vi "一体站氨氮总磷流程质控自动启动.vi"(6 "CODMn量程切换":enum32{"H", "L", "AUTO"}(ring)=enum."AUTO", 8 "总磷量程切换":enum32{"H", "L", "AUTO"}(ring)=enum."AUTO", 9 "总氮量程切换":enum32{"H", "L", "AUTO"}(ring)=enum."AUTO", 10 "氨氮量程切换":enum32{"H", "L", "AUTO"}(ring)=enum."AUTO", 11 "参数":T1={"是否启用仪器"=FALSE, "CODMn"={"启动测量模式"={"测量模式"=enum."水样测量"}, "确定按钮"=TRUE}, "启动模块"={"氨氮"=FALSE, "总磷"=FALSE, "总氮"=FALSE, "CODMn"=FALSE, "CODCr"=FALSE}, "常规启动"=FALSE, "直接启动"=FALSE}) -> ()   [LabVIEW 2016, in "质控单元.lvlib"]
panel:
  out "枚举 2":enum16{"初始化", "采配水启动", "等待", "配水", "排水", "结束"}(ring)
  out "枚举":enum16{"初始化", "采配水启动", "等待", "配水", "排水", "结束"}(ring)
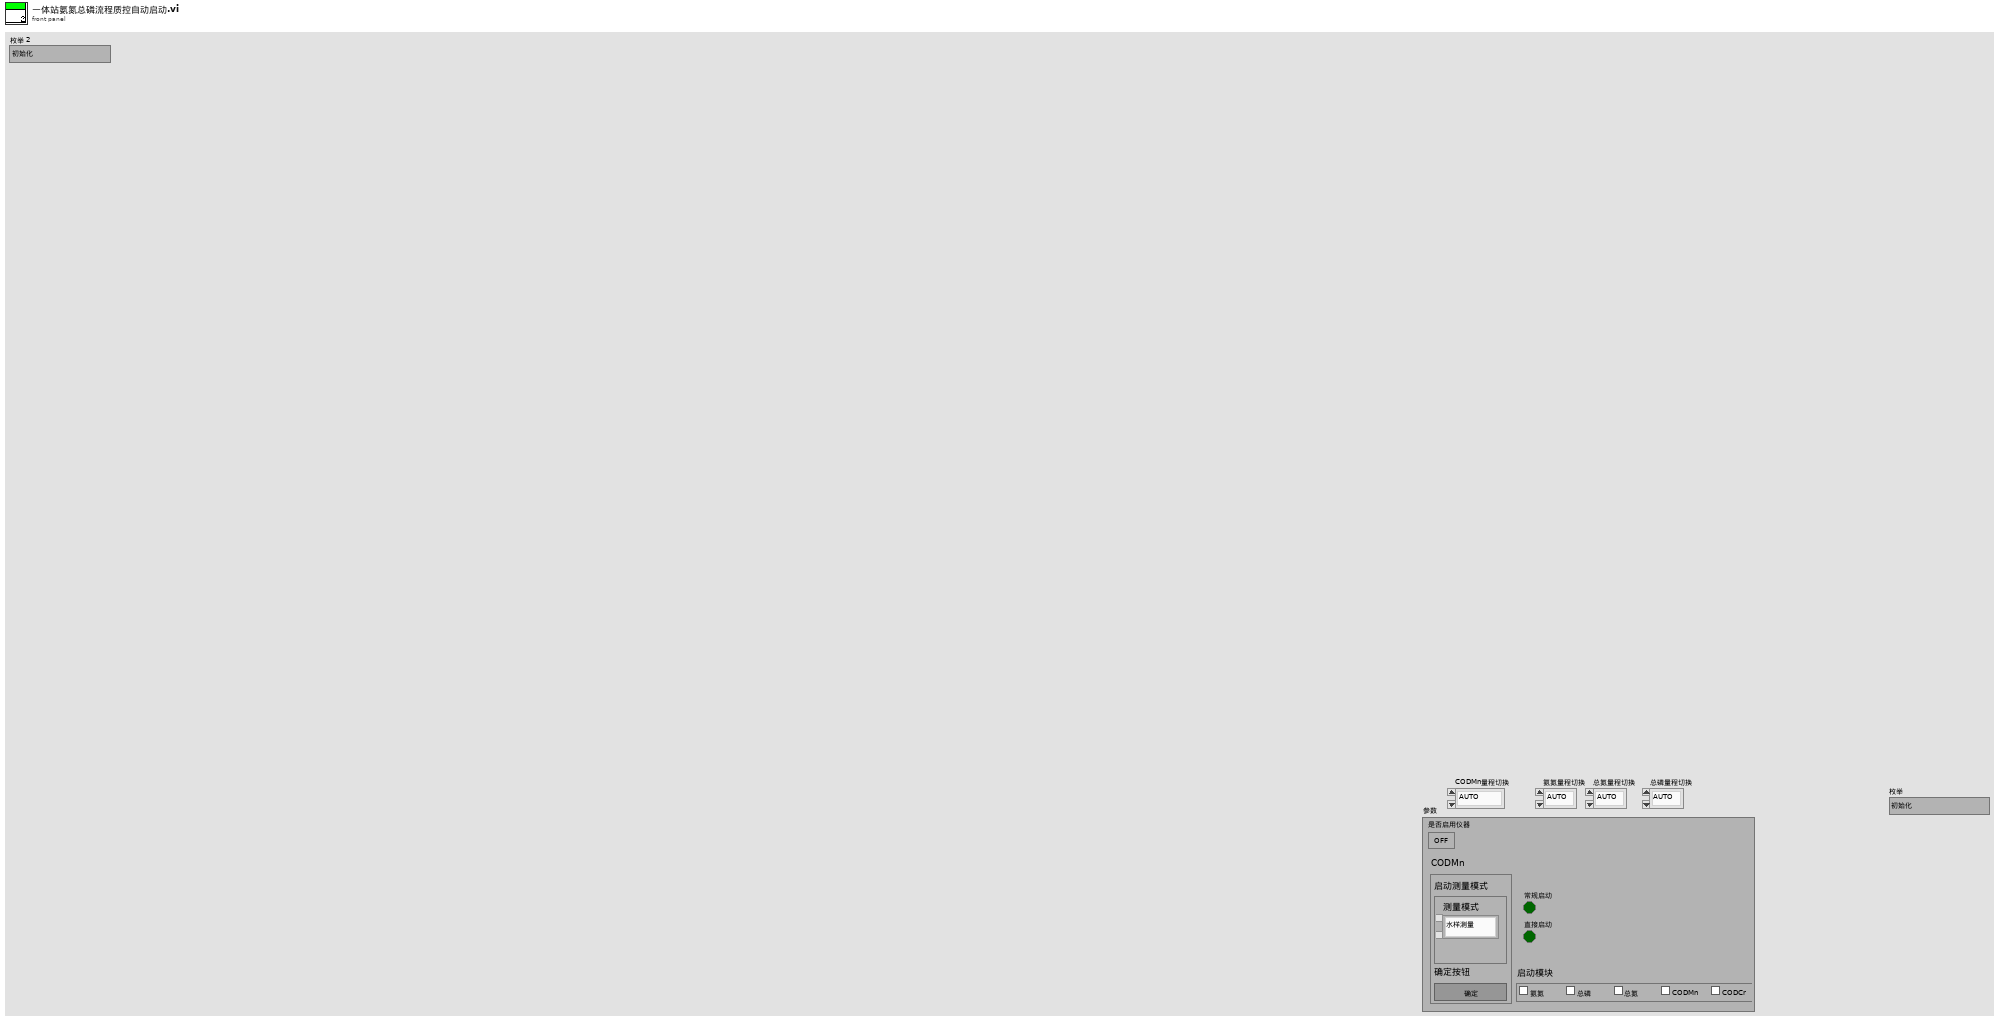
[diagram p1: front panel]
types:
  T1 = cluster{"是否启用仪器":bool, "CODMn":cluster{"启动测量模式":cluster{"测量模式":enum16{"水样测量", "标样核查", "加标回收", "平行样", "校零", "校标"}}, "确定按钮":bool}, "启动模块":cluster{"氨氮":bool, "总磷":bool, "总氮":bool, "CODMn":bool, "CODCr":bool}, "常规启动":bool, "直接启动":bool}
  T2 = cluster{"命令":string, cluster{"starting address":u16, "holding register value":u16}}
  T3 = cluster{"R0":i16, "R1":i16, "R2":i16, "R3":i16, "R4":i16, "R5":i16, "R6":i16, "R7":i16, "R8":i16, "R9":i16, "R10":i16, "R11":i16, "R12":i16, "R13":i16, "R14":i16, "R15":i16, "R16":i16, "R17":i16, "R18":i16, "R19":i16, "R20":i16, "R21":i16, "R22":i16, "R23":i16, "R24":i16, "R25":i16, "R26":i16, "R27":i16, "R28":i16, "R29":i16, "R30":i16, "R31":i16, "R32":i16, "R33":i16, "R34":i16, "R35":i16, "R36":i16, "R37":i16, "R38":i16, "R39":i16, "R40":i16, "R41":i16, "R42":i16, "R43":i16, "R44":i16, "R45":i16, "R46":i16, "R47":i16, "R48":i16, "R49":i16, "R50":i16, "R51":i16, "R52":i16, "R53":i16, "R54":i16, "R55":i16, "R56":i16}
  T4 = enum32{"Bad", "Idle", "Run top level", "Running"}
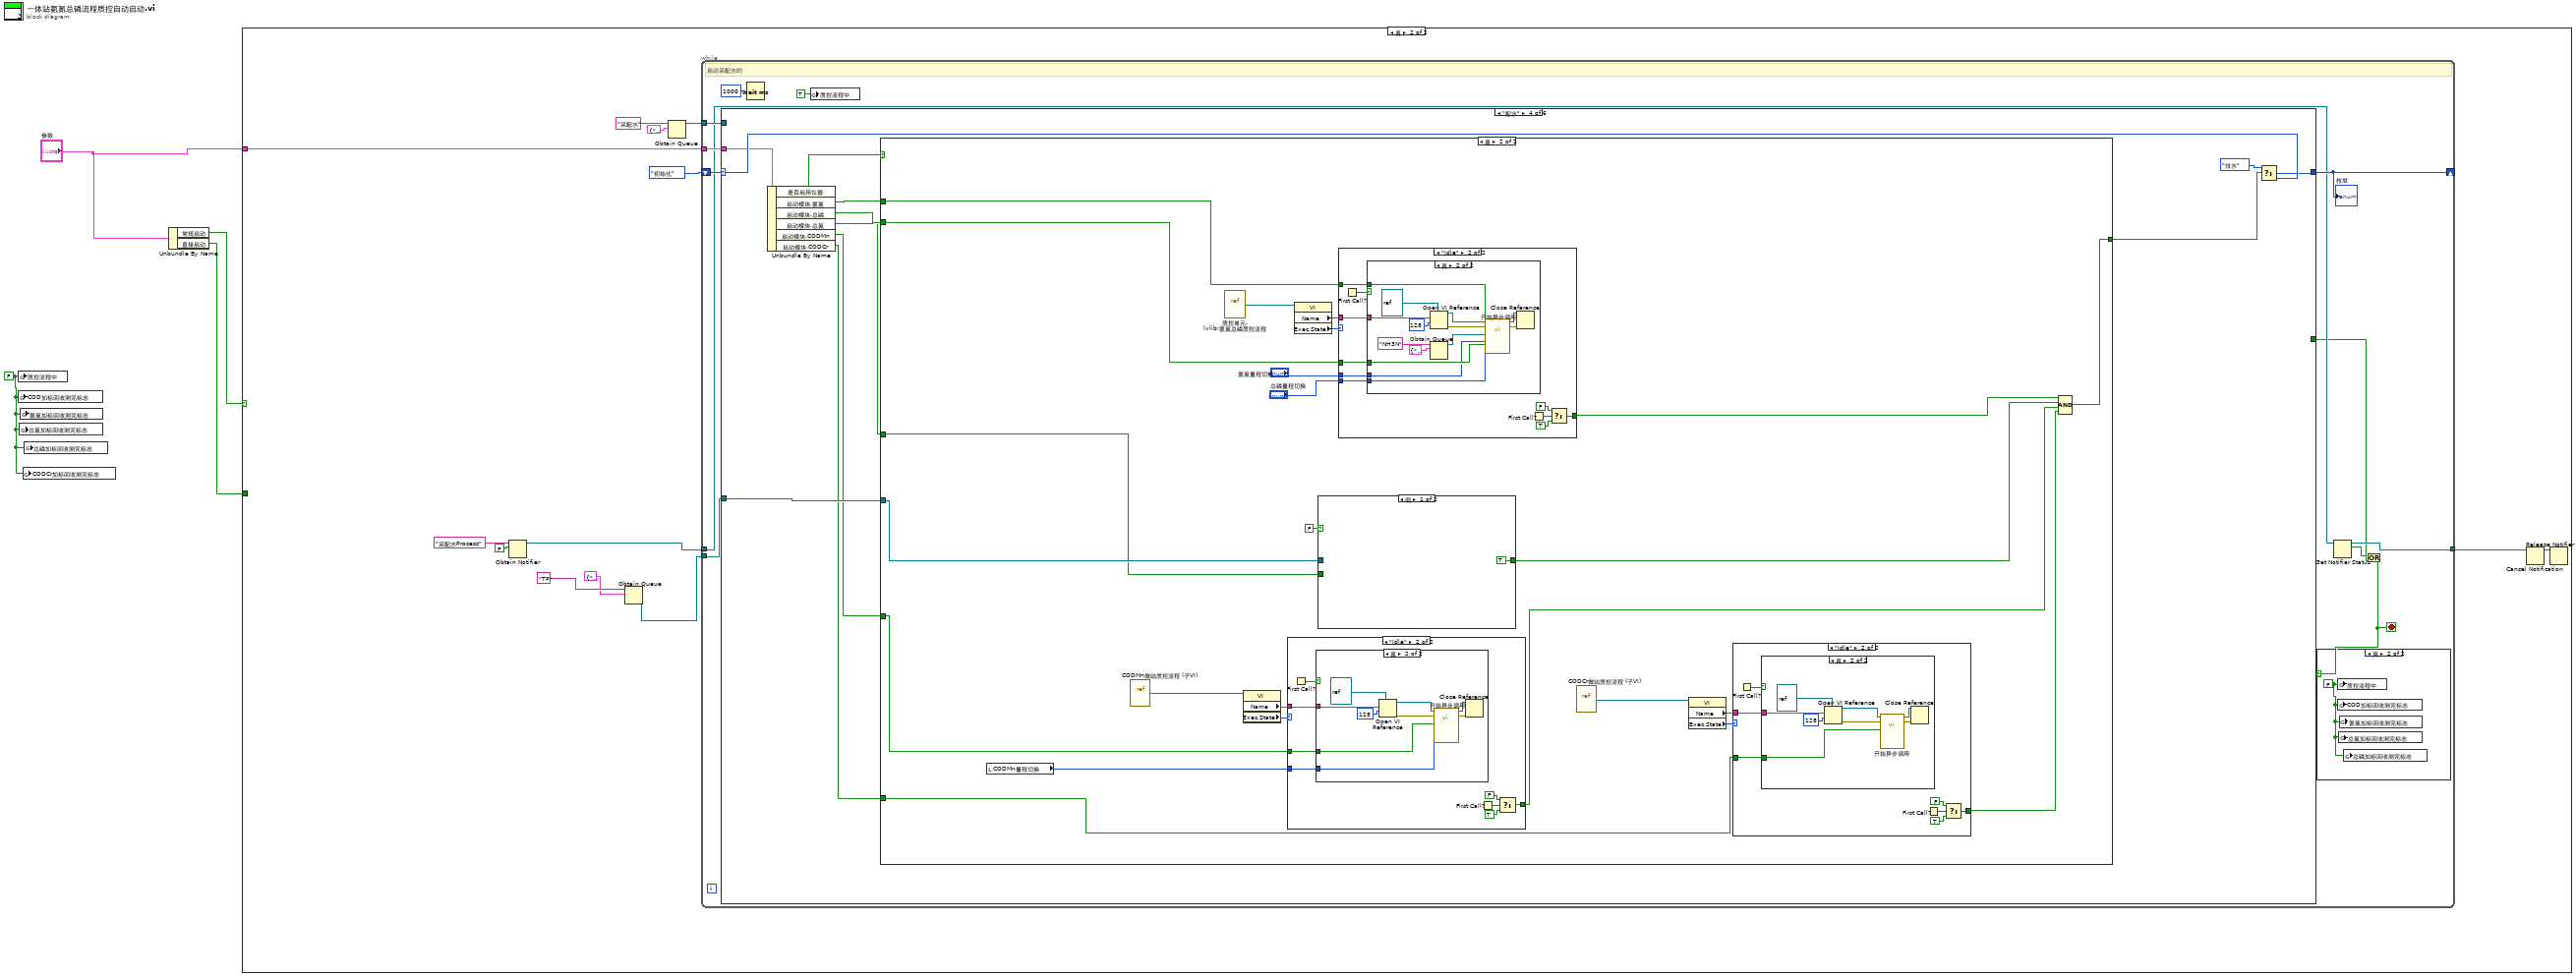
[diagram p0: block diagram]
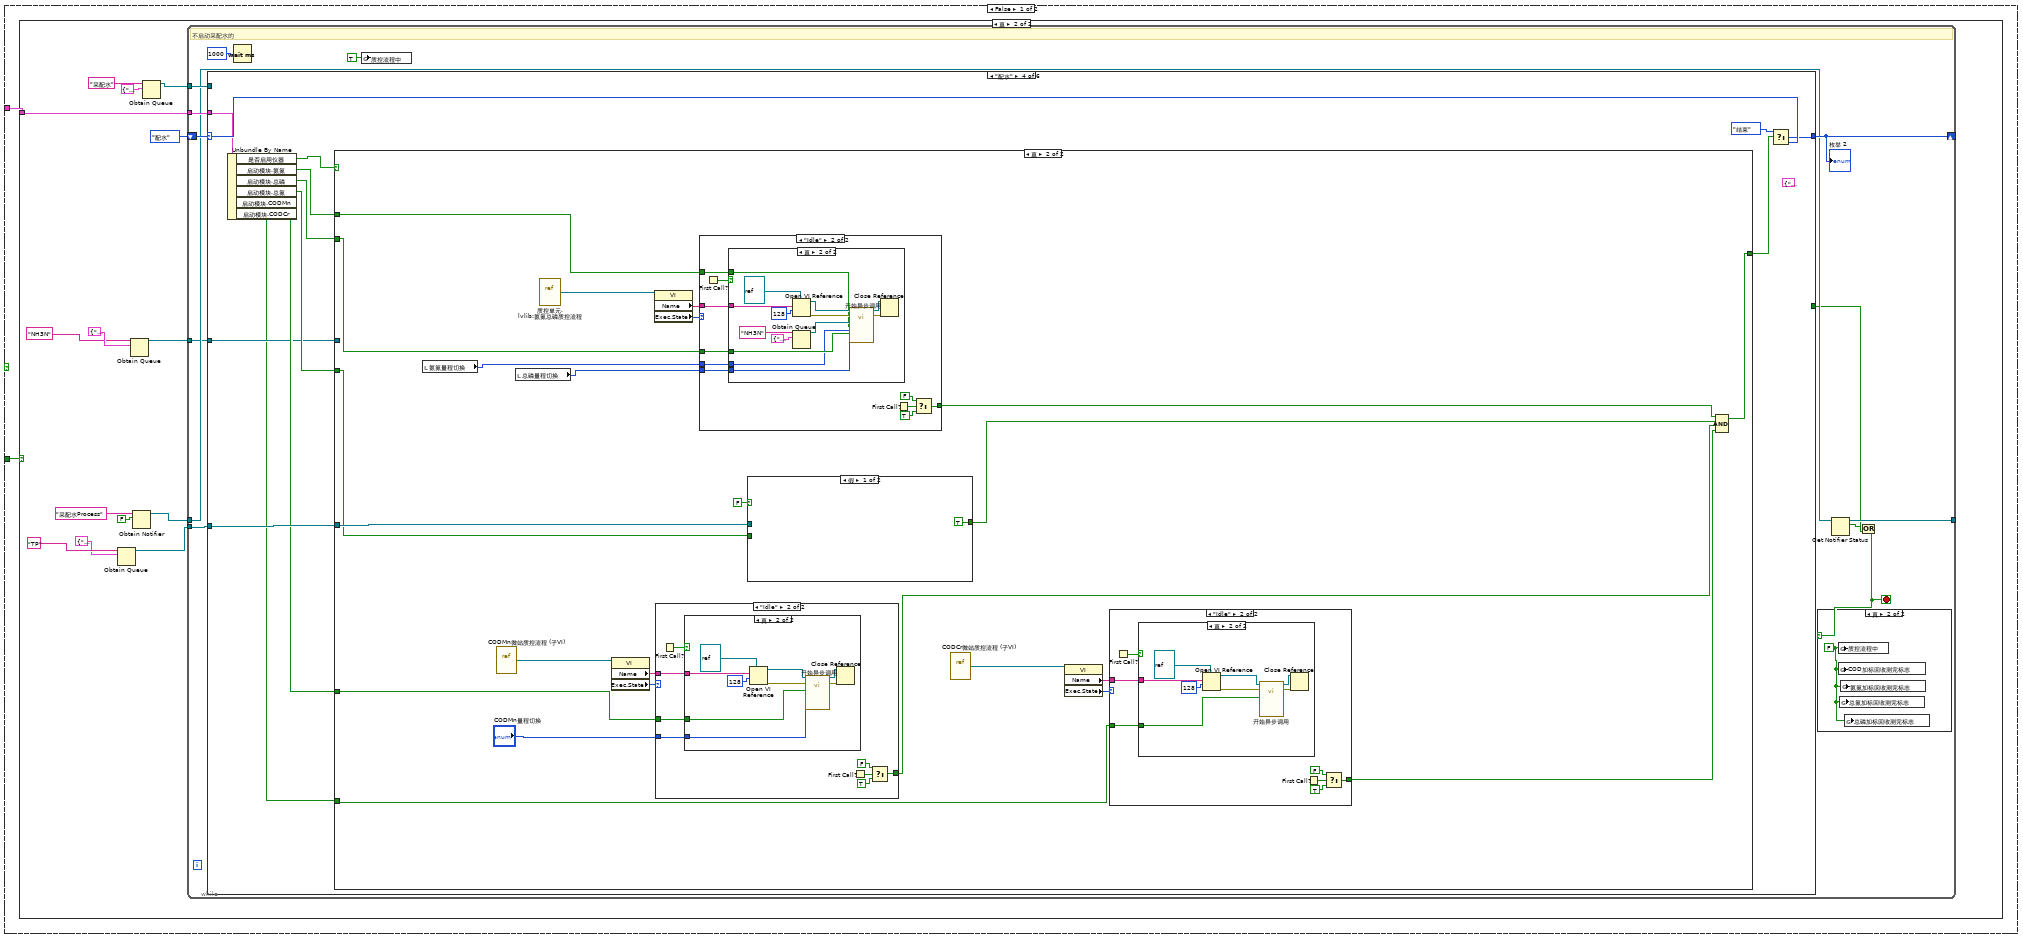
[diagram p2: hidden frame]
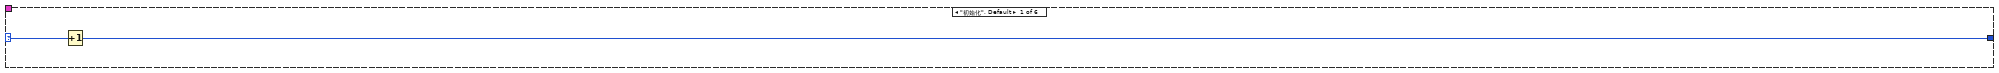
[diagram p5: hidden frame]
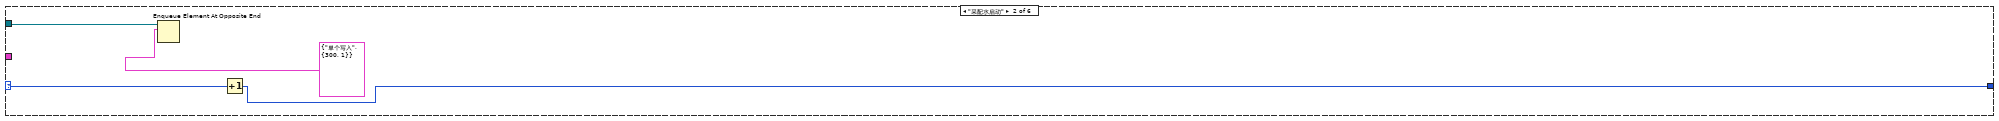
[diagram p6: hidden frame]
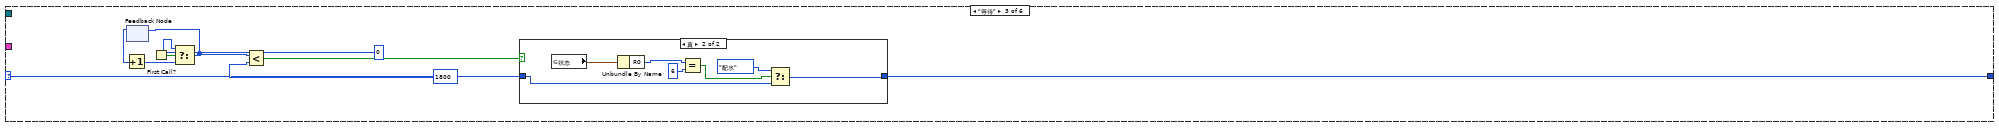
[diagram p7: hidden frame]
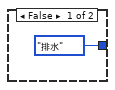
[diagram p8: hidden frame]
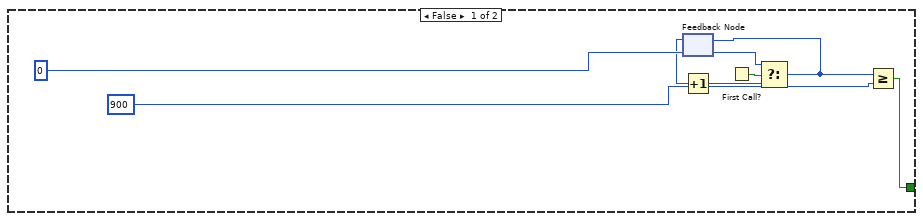
[diagram p9: hidden frame]
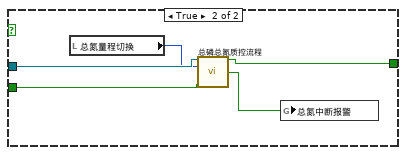
[diagram p16: hidden frame]
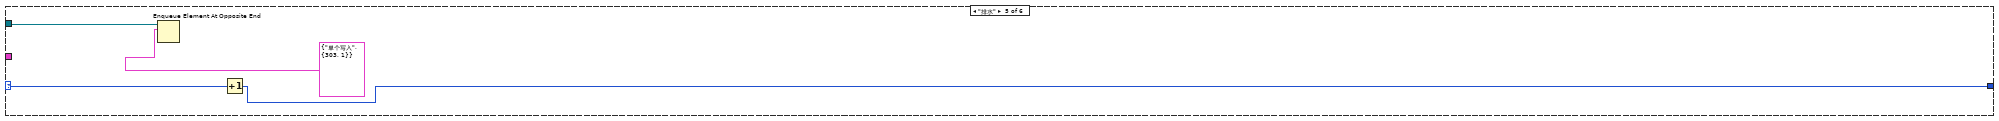
[diagram p17: hidden frame]
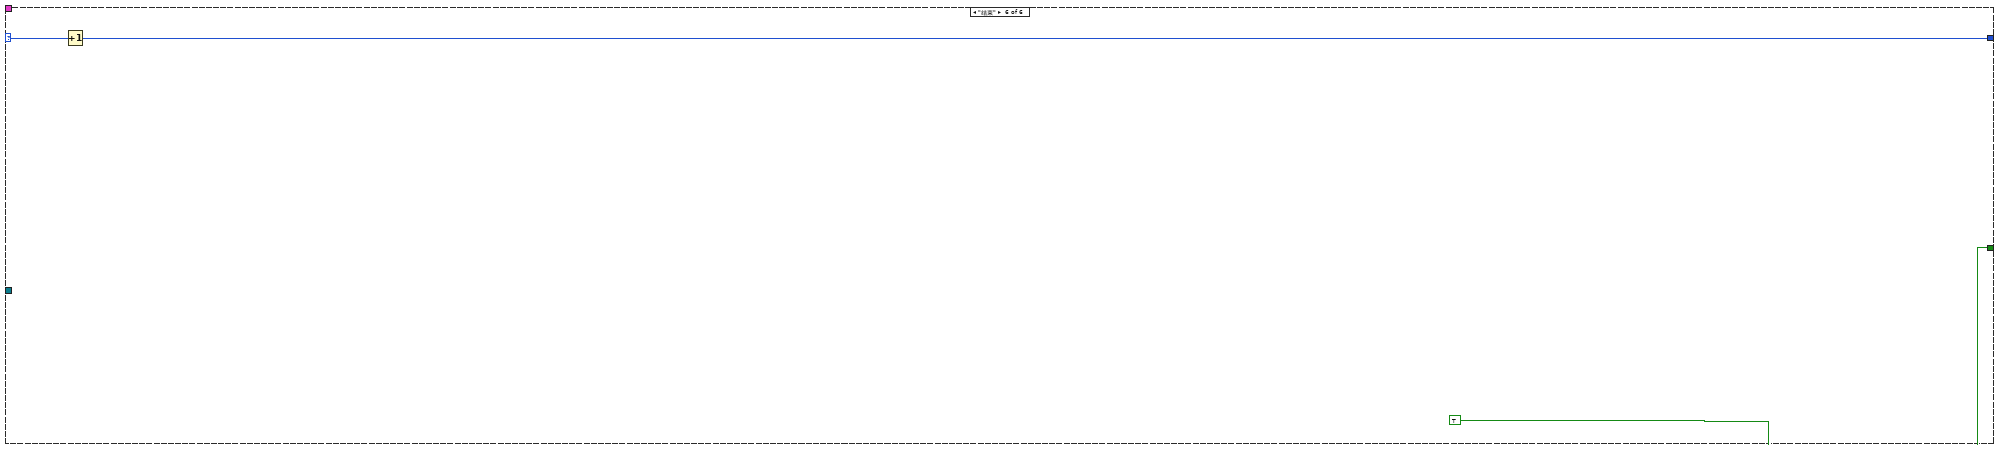
[diagram p18: hidden frame]
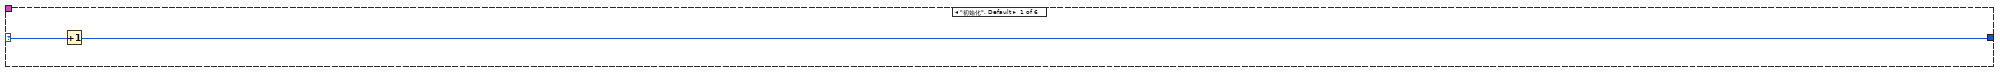
[diagram p20: hidden frame]
diagram:
  w2 = FALSE ("质控流程中")
  n1 = global write "质控测完标志全局 1.vi" "质控流程中"(w2) -> ()
  n2 = global write "质控测完标志全局 1.vi" "COD加标回收测完标志"(w2) -> ()
  n3 = global write "质控测完标志全局 1.vi" "总氮加标回收测完标志"(w2) -> ()
  n4 = global write "质控测完标志全局 1.vi" "氨氮加标回收测完标志"(w2) -> ()
  n5 = global write "质控测完标志全局 1.vi" "CODCr加标回收测完标志"(w2) -> ()
  n6 = global write "质控测完标志全局 1.vi" "总磷加标回收测完标志"(w2) -> ()
  n7 = Unbundle By Name("参数") -> ("常规启动"=w1:bool, "直接启动"=w3:bool)
  n8 = case shown="真" w1 {
    tunnel: "参数" -> [w5 w171]
    tunnel: w3 -> [w6 _]
    frame False {
      n9 = case shown="真" w6 {
        tunnel: w5 -> [_ w19]
        frame False {
        }
        frame True {
          n10 = Obtain Queue(name (unnamed)="TP" ("名称（未命名）"), element data type=cluster{"命令":string, "data":variant} {"命令"="", "data"=variant}) -> (queue out=w10:refnum<queue>)  [unwired: 3 in, 2 out]
          n11 = Obtain Queue(name (unnamed)="NH3N" ("名称（未命名）"), element data type=cluster{"命令":string, "data":variant} {"命令"="", "data"=variant}) -> (queue out=w7:refnum<queue>)  [unwired: 3 in, 2 out]
          n12 = Obtain Notifier(name (unnamed)="采配水Process" ("名称（未命名）"), notification data type=FALSE) -> (notifier out=w13:refnum<notifier>)  [unwired: 2 in, 2 out]
          n13 = Obtain Queue(name (unnamed)="采配水" ("名称（未命名）"), element data type=cluster{"命令":string, "数据":variant} {"命令"="", "数据"=variant}) -> (queue out=w16:refnum<queue>)  [unwired: 3 in, 2 out]
          n14 = while {
            tunnel: w16 -> [w33]
            shift-right: [w31] -> _
            shift-left: enum16{"初始化", "采配水启动", "等待", "配水", "排水", "结束"}."配水" ("枚举") -> [w32]
            tunnel: w10 -> [w29]
            tunnel: w19 -> [w28]
            tunnel: w13 -> [w27]
            tunnel: [w26] -> _
            tunnel: w7 -> [w23]
            stop <- w22 stop-if-true
            # "不启动采配水的"
            n15 = case shown="\"配水\"" w32 {
              selector: w32 -> [w36 w38 w47 w69 w165 w170]
              tunnel: w33 -> [_ w39 _ _ w166 _]
              tunnel: [w35 w37 w46 w68 w164 w169] -> w31
              tunnel: [_ _ _ _ _ TRUE] -> w25
              tunnel: w29 -> [_ _ _ w67 _ _]
              tunnel: w28 -> [_ _ _ w64 _ _]
              tunnel: w23 -> [_ _ _ w59 _ _]
              frame "初始化", Default {
                n16 = Increment(x=w36) -> (x+1=w35:enum16{"初始化", "采配水启动", "等待", "配水", "排水", "结束"})
              }
              frame "采配水启动" {
                n17 = Enqueue Element At Opposite End(queue=w39, element=T2 {"命令"="单个写入", {"starting address"=300, "holding register value"=1}} ("元素")) -> ()  [unwired: 2 in, 3 out]
                n18 = Increment(x=w38) -> (x+1=w37:enum16{"初始化", "采配水启动", "等待", "配水", "排水", "结束"})
              }
              frame "等待" {
                n19 = feedback #1() -> (w43:i32)  [unwired: 1 in]
                n20 = Increment(x=w43) -> (x+1=w42:i32)
                n21 = First Call?() -> (First Call?: T/F=w44:bool)
                n22 = Select(t=0, s=w44, f=w42) -> (s? t:f=w41:i32)
                n23 = feedback-in #1(w41) -> ()
                n24 = Less?(x=w41, y=1800) -> (x < y?=w48:bool)
                n25 = case shown="真" w48 {
                  tunnel: w47 -> [_ w53]
                  tunnel: [enum16{"初始化", "采配水启动", "等待", "配水", "排水", "结束"}."排水" ("枚举") w52] -> w46
                  frame False {
                  }
                  frame True {
                    n26 = global read "与采配水交互全局.vi" "状态"() -> (w51:T3)
                    n27 = Unbundle By Name(w51) -> ("R0"=w57:i16)
                    n28 = Equal?(x=w57, y=i16 6) -> (x = y?=w55:bool)
                    n29 = Select(t=enum16{"初始化", "采配水启动", "等待", "配水", "排水", "结束"}."配水" ("枚举"), s=w55, f=w53) -> (s? t:f=w52:enum16{"初始化", "采配水启动", "等待", "配水", "排水", "结束"})
                  }
                }
              }
              frame "配水" {
                (unwired) cluster{"命令":string, "data":variant} {"命令"="启动", "data"=variant(cluster{"站号":u16, "控制命令输出":u16[]} {"站号"=1, "控制命令输出"=[256, 0]})} ("元素")
                n30 = Unbundle By Name(w64) -> ("是否启用仪器"=w66:bool, "启动模块.氨氮"=w62:bool, "启动模块.总磷"=w63:bool, "启动模块.总氮"=w60:bool, "启动模块.CODMn"=w61:bool, "启动模块.CODCr"=w58:bool)
                n31 = case shown="真" w66 {
                  tunnel: w67 -> [_ w100]
                  tunnel: [w71 w101] -> w65
                  tunnel: w63 -> [_ w90]
                  tunnel: w62 -> [_ w93]
                  tunnel: w61 -> [_ w83]
                  tunnel: w60 -> [_ w99]
                  tunnel: w59 -> [_ _]
                  tunnel: w58 -> [_ w81]
                  frame False {
                    n32 = feedback #2() -> (w75:i32)  [unwired: 1 in]
                    n33 = Increment(x=w75) -> (x+1=w74:i32)
                    n34 = First Call?() -> (First Call?: T/F=w76:bool)
                    n35 = Select(t=0, s=w76, f=w74) -> (s? t:f=w72:i32)
                    n36 = feedback-in #2(w72) -> ()
                    n37 = Greater Or Equal?(x=w72, y=900) -> (x >= y?=w71:bool)
                  }
                  frame True {
                    n38 = local read "氨氮量程切换"() -> (w92:enum32{"H", "L", "AUTO"})
                    n39 = vi-ref "CODMn微站质控流程 (子VI).vi"() -> (w89:refnum<vi>)
                    n40 = local read "总磷量程切换"() -> (w91:enum32{"H", "L", "AUTO"})
                    n41 = vi-ref "质控单元.lvlib:氨氮总磷质控流程.vi"() -> (w96:refnum<vi>)
                    n42 = property class="VI"(reference=w89) -> ("Name"=w88:string, "Exec.State"=w87:T4)  [unwired: 1 in, 2 out]
                    n43 = property class="VI"(reference=w96) -> ("Name"=w95:string, "Exec.State"=w94:T4)  [unwired: 1 in, 2 out]
                    n44 = case shown="\"Idle\"" w87 {
                      tunnel: w88 -> [_ w124]
                      tunnel: [_ w119] -> w79
                      tunnel: w83 -> [_ w118]
                      tunnel: "CODMn量程切换" -> [_ w117]
                      frame "Bad", Default {
                      }
                      frame "Idle" {
                        n45 = First Call?() -> (First Call?: T/F=w123:bool)
                        n46 = case shown="真" w123 {
                          tunnel: w124 -> [_ w133]
                          tunnel: w118 -> [_ w126]
                          tunnel: w117 -> [_ w125]
                          frame False {
                          }
                          frame True {
                            n47 = Open VI Reference(type specifier VI Refnum (for type only)=refnum<vi> refnum ("类型说明符VI引用句柄（仅用于类型）"), vi path=w133, options=128 ("选项")) -> (vi reference=w127:refnum<vi>, error out=w130:errorcluster)  [unwired: 3 in]
                            n48 = call-by-ref "开始异步调用"(reference=w127, error in=w130, "CODMn量程切换"=w125, "COD"=w126) -> (reference out=w132:refnum<vi>, error out=w131:errorcluster)  [unwired: 8 in, 2 out]
                            n49 = Close Reference(reference=w132, error in (no error)=w131) -> ()  [unwired: 1 out]
                          }
                        }
                        n50 = First Call?() -> (First Call?: T/F=w122:bool)
                        n51 = Select(t=FALSE, s=w122, f=TRUE) -> (s? t:f=w119:bool)
                      }
                    }
                    n52 = case shown="\"Idle\"" w94 {
                      tunnel: w95 -> [_ w143]
                      tunnel: [_ w138] -> w78
                      tunnel: w93 -> [_ w137]
                      tunnel: w90 -> [_ w136]
                      tunnel: w92 -> [_ w135]
                      tunnel: w91 -> [_ w134]
                      frame "Bad", Default {
                      }
                      frame "Idle" {
                        n53 = First Call?() -> (First Call?: T/F=w142:bool)
                        n54 = case shown="真" w142 {
                          tunnel: w143 -> [_ w156]
                          tunnel: w137 -> [_ w147]
                          tunnel: w136 -> [_ w146]
                          tunnel: w135 -> [_ w145]
                          tunnel: w134 -> [_ w144]
                          frame False {
                          }
                          frame True {
                            n55 = Obtain Queue(name (unnamed)="NH3N" ("名称（未命名）"), element data type=cluster{"命令":string, "data":variant} {"命令"="", "data"=variant}) -> (queue out=w148:refnum<queue>)  [unwired: 3 in, 2 out]
                            n56 = Open VI Reference(type specifier VI Refnum (for type only)=refnum<vi> refnum ("类型说明符VI引用句柄（仅用于类型）"), vi path=w156, options=128 ("选项")) -> (vi reference=w157:refnum<vi>, error out=w153:errorcluster)  [unwired: 3 in]
                            n57 = call-by-ref "开始异步调用"(reference=w157, error in=w153, "队列输入"=w148, "氨氮"=w147, "氨氮量程切换"=w145, "总磷"=w146, "总磷量程切换"=w144) -> (reference out=w155:refnum<vi>, error out=w154:errorcluster)  [unwired: 8 in, 3 out]
                            n58 = Close Reference(reference=w155, error in (no error)=w154) -> ()  [unwired: 1 out]
                          }
                        }
                        n59 = First Call?() -> (First Call?: T/F=w141:bool)
                        n60 = Select(t=FALSE, s=w141, f=TRUE) -> (s? t:f=w138:bool)
                      }
                    }
                    n61 = case shown="假" FALSE {
                      tunnel: w100 -> [_ w163]
                      tunnel: w99 -> [_ w162]
                      tunnel: [TRUE ("布尔") w161] -> w98
                      frame False {
                      }
                      frame True {
                        n62 = local read "总氮量程切换"() -> (w160:enum32{"H", "L", "AUTO"})
                        n63 = call "总磷总氮质控流程.vi"("队列输入TP"=w163, "总氮量程切换"=w160, "总氮"=w162) -> ("布尔"=w161:bool, "总氮中断报警"=w159:bool)  [unwired: 10 in, 1 out]
                        n64 = global write "质控中断报警全局.vi" "总氮中断报警"(w159) -> ()
                      }
                    }
                    n65 = vi-ref "CODCr微站质控流程 (子VI).vi"() -> (w84:refnum<vi>)
                    n66 = property class="VI"(reference=w84) -> ("Name"=w85:string, "Exec.State"=w86:T4)  [unwired: 1 in, 2 out]
                    n67 = case shown="\"Idle\"" w86 {
                      tunnel: w85 -> [_ w108]
                      tunnel: [_ w103] -> w80
                      tunnel: w81 -> [_ w102]
                      frame "Bad", Default {
                      }
                      frame "Idle" {
                        n68 = First Call?() -> (First Call?: T/F=w107:bool)
                        n69 = case shown="真" w107 {
                          tunnel: w108 -> [_ w116]
                          tunnel: w102 -> [_ w109]
                          frame False {
                          }
                          frame True {
                            n70 = Open VI Reference(type specifier VI Refnum (for type only)=refnum<vi> refnum ("类型说明符VI引用句柄（仅用于类型）"), vi path=w116, options=128 ("选项")) -> (vi reference=w110:refnum<vi>, error out=w113:errorcluster)  [unwired: 3 in]
                            n71 = call-by-ref "开始异步调用"(reference=w110, error in=w113, "COD"=w109) -> (reference out=w115:refnum<vi>, error out=w114:errorcluster)  [unwired: 9 in, 2 out]
                            n72 = Close Reference(reference=w115, error in (no error)=w114) -> ()  [unwired: 1 out]
                          }
                        }
                        n73 = First Call?() -> (First Call?: T/F=w106:bool)
                        n74 = Select(t=FALSE, s=w106, f=TRUE) -> (s? t:f=w103:bool)
                      }
                    }
                    n75 = Compound Arithmetic op=AND ("复合运算")(w78, w98, w79, w80) -> (w101:bool)
                  }
                }
                n76 = Select(t=enum16{"初始化", "采配水启动", "等待", "配水", "排水", "结束"}."结束" ("枚举"), s=w65, f=w69) -> (s? t:f=w68:enum16{"初始化", "采配水启动", "等待", "配水", "排水", "结束"})
              }
              frame "排水" {
                n77 = Enqueue Element At Opposite End(queue=w166, element=T2 {"命令"="单个写入", {"starting address"=303, "holding register value"=1}} ("元素")) -> ()  [unwired: 2 in, 3 out]
                n78 = Increment(x=w165) -> (x+1=w164:enum16{"初始化", "采配水启动", "等待", "配水", "排水", "结束"})
              }
              frame "结束" {
                n79 = Increment(x=w170) -> (x+1=w169:enum16{"初始化", "采配水启动", "等待", "配水", "排水", "结束"})
              }
            }
            "枚举 2" <- w31
            n80 = Wait (ms)(milliseconds to wait=u32 1000 ("等待时间（毫秒）")) -> ()  [unwired: 1 out]
            n81 = global write "质控测完标志全局 1.vi" "质控流程中"(TRUE ("质控流程中")) -> ()
            n82 = Get Notifier Status(notifier=w27) -> (notifier out=w26:refnum<notifier>, current notification=w24:bool)  [unwired: 1 in, 3 out]
            n83 = Or(x=w24, y=w25) -> (x .or. y?=w22:bool)
            n84 = case shown="真" w22 {
              frame False {
              }
              frame True {
                w34 = FALSE ("质控流程中")
                n85 = global write "质控测完标志全局 1.vi" "质控流程中"(w34) -> ()
                n86 = global write "质控测完标志全局 1.vi" "COD加标回收测完标志"(w34) -> ()
                n87 = global write "质控测完标志全局 1.vi" "总氮加标回收测完标志"(w34) -> ()
                n88 = global write "质控测完标志全局 1.vi" "氨氮加标回收测完标志"(w34) -> ()
                n89 = global write "质控测完标志全局 1.vi" "总磷加标回收测完标志"(w34) -> ()
              }
            }
          }
        }
      }
    }
    frame True {
      n90 = Obtain Notifier(name (unnamed)="采配水Process" ("名称（未命名）"), notification data type=FALSE) -> (notifier out=w174:refnum<notifier>)  [unwired: 2 in, 2 out]
      n91 = Obtain Queue(name (unnamed)="TP" ("名称（未命名）"), element data type=cluster{"命令":string, "data":variant} {"命令"="", "data"=variant}) -> (queue out=w177:refnum<queue>)  [unwired: 3 in, 2 out]
      n92 = Obtain Queue(name (unnamed)="采配水" ("名称（未命名）"), element data type=cluster{"命令":string, "数据":variant} {"命令"="", "数据"=variant}) -> (queue out=w181:refnum<queue>)  [unwired: 3 in, 2 out]
      n93 = while {
        tunnel: w181 -> [w195]
        shift-right: [w193] -> _
        shift-left: enum16{"初始化", "采配水启动", "等待", "配水", "排水", "结束"}."初始化" ("枚举") -> [w194]
        tunnel: w177 -> [w191]
        tunnel: w171 -> [w190]
        tunnel: w174 -> [w189]
        tunnel: [w188] -> w173
        stop <- w185 stop-if-true
        # "启动采配水的"
        n94 = case shown="\"配水\"" w194 {
          selector: w194 -> [w198 w200 w209 w230 w326 w331]
          tunnel: w195 -> [_ w201 _ _ w327 _]
          tunnel: [w197 w199 w208 w229 w325 w330] -> w193
          tunnel: [_ _ _ _ _ TRUE] -> w187
          tunnel: w191 -> [_ _ _ w228 _ _]
          tunnel: w190 -> [_ _ _ w225 _ _]
          frame "初始化", Default {
            n95 = Increment(x=w198) -> (x+1=w197:enum16{"初始化", "采配水启动", "等待", "配水", "排水", "结束"})
          }
          frame "采配水启动" {
            n96 = Enqueue Element At Opposite End(queue=w201, element=T2 {"命令"="单个写入", {"starting address"=300, "holding register value"=1}} ("元素")) -> ()  [unwired: 2 in, 3 out]
            n97 = Increment(x=w200) -> (x+1=w199:enum16{"初始化", "采配水启动", "等待", "配水", "排水", "结束"})
          }
          frame "等待" {
            n98 = feedback #3() -> (w205:i32)  [unwired: 1 in]
            n99 = Increment(x=w205) -> (x+1=w204:i32)
            n100 = First Call?() -> (First Call?: T/F=w206:bool)
            n101 = Select(t=0, s=w206, f=w204) -> (s? t:f=w203:i32)
            n102 = feedback-in #3(w203) -> ()
            n103 = Less?(x=w203, y=1800) -> (x < y?=w210:bool)
            n104 = case shown="真" w210 {
              tunnel: w209 -> [_ w215]
              tunnel: [enum16{"初始化", "采配水启动", "等待", "配水", "排水", "结束"}."排水" ("枚举") w214] -> w208
              frame False {
              }
              frame True {
                n105 = global read "与采配水交互全局.vi" "状态"() -> (w213:T3)
                n106 = Unbundle By Name(w213) -> ("R0"=w219:i16)
                n107 = Equal?(x=w219, y=i16 6) -> (x = y?=w217:bool)
                n108 = Select(t=enum16{"初始化", "采配水启动", "等待", "配水", "排水", "结束"}."配水" ("枚举"), s=w217, f=w215) -> (s? t:f=w214:enum16{"初始化", "采配水启动", "等待", "配水", "排水", "结束"})
              }
            }
          }
          frame "配水" {
            n109 = Unbundle By Name(w225) -> ("是否启用仪器"=w227:bool, "启动模块.氨氮"=w223:bool, "启动模块.总磷"=w224:bool, "启动模块.总氮"=w221:bool, "启动模块.CODMn"=w222:bool, "启动模块.CODCr"=w220:bool)
            n110 = case shown="真" w227 {
              tunnel: w228 -> [_ w261]
              tunnel: [w232 w262] -> w226
              tunnel: w224 -> [_ w253]
              tunnel: w223 -> [_ w254]
              tunnel: w222 -> [_ w246]
              tunnel: w221 -> [_ w260]
              tunnel: w220 -> [_ w240]
              frame False {
                n111 = feedback #4() -> (w236:i32)  [unwired: 1 in]
                n112 = Increment(x=w236) -> (x+1=w235:i32)
                n113 = First Call?() -> (First Call?: T/F=w237:bool)
                n114 = Select(t=0, s=w237, f=w235) -> (s? t:f=w233:i32)
                n115 = feedback-in #4(w233) -> ()
                n116 = Greater Or Equal?(x=w233, y=900) -> (x >= y?=w232:bool)
              }
              frame True {
                n117 = local read "CODMn量程切换"() -> (w244:enum32{"H", "L", "AUTO"})
                n118 = vi-ref "CODMn微站质控流程 (子VI).vi"() -> (w249:refnum<vi>)
                n119 = vi-ref "质控单元.lvlib:氨氮总磷质控流程.vi"() -> (w257:refnum<vi>)
                n120 = property class="VI"(reference=w249) -> ("Name"=w248:string, "Exec.State"=w247:T4)  [unwired: 1 in, 2 out]
                n121 = case shown="\"Idle\"" w247 {
                  tunnel: w248 -> [_ w285]
                  tunnel: [_ w280] -> w245
                  tunnel: w246 -> [_ w279]
                  tunnel: w244 -> [_ w278]
                  frame "Bad", Default {
                  }
                  frame "Idle" {
                    n122 = First Call?() -> (First Call?: T/F=w284:bool)
                    n123 = case shown="真" w284 {
                      tunnel: w285 -> [_ w294]
                      tunnel: w279 -> [_ w287]
                      tunnel: w278 -> [_ w286]
                      frame False {
                      }
                      frame True {
                        n124 = Open VI Reference(type specifier VI Refnum (for type only)=refnum<vi> refnum ("类型说明符VI引用句柄（仅用于类型）"), vi path=w294, options=128 ("选项")) -> (vi reference=w288:refnum<vi>, error out=w291:errorcluster)  [unwired: 3 in]
                        n125 = call-by-ref "开始异步调用"(reference=w288, error in=w291, "CODMn量程切换"=w286, "COD"=w287) -> (reference out=w293:refnum<vi>, error out=w292:errorcluster)  [unwired: 8 in, 2 out]
                        n126 = Close Reference(reference=w293, error in (no error)=w292) -> ()  [unwired: 1 out]
                      }
                    }
                    n127 = First Call?() -> (First Call?: T/F=w283:bool)
                    n128 = Select(t=FALSE, s=w283, f=TRUE) -> (s? t:f=w280:bool)
                  }
                }
                n129 = property class="VI"(reference=w257) -> ("Name"=w256:string, "Exec.State"=w255:T4)  [unwired: 1 in, 2 out]
                n130 = case shown="假" FALSE {
                  tunnel: w261 -> [_ w324]
                  tunnel: w260 -> [_ w323]
                  tunnel: [TRUE ("布尔") w322] -> w259
                  frame False {
                  }
                  frame True {
                    n131 = call "总磷总氮质控流程.vi"("队列输入TP"=w324, "总氮量程切换"="总氮量程切换", "总氮"=w323) -> ("布尔"=w322:bool, "总氮中断报警"=w320:bool)  [unwired: 10 in, 1 out]
                    n132 = global write "质控中断报警全局.vi" "总氮中断报警"(w320) -> ()
                  }
                }
                n133 = case shown="\"Idle\"" w255 {
                  tunnel: w256 -> [_ w304]
                  tunnel: [_ w299] -> w252
                  tunnel: w254 -> [_ w298]
                  tunnel: w253 -> [_ w297]
                  tunnel: "氨氮量程切换" -> [_ w296]
                  tunnel: "总磷量程切换" -> [_ w295]
                  frame "Bad", Default {
                  }
                  frame "Idle" {
                    n134 = First Call?() -> (First Call?: T/F=w303:bool)
                    n135 = case shown="真" w303 {
                      tunnel: w304 -> [_ w317]
                      tunnel: w298 -> [_ w308]
                      tunnel: w297 -> [_ w307]
                      tunnel: w296 -> [_ w306]
                      tunnel: w295 -> [_ w305]
                      frame False {
                      }
                      frame True {
                        n136 = Obtain Queue(name (unnamed)="NH3N" ("名称（未命名）"), element data type=cluster{"命令":string, "data":variant} {"命令"="", "data"=variant}) -> (queue out=w309:refnum<queue>)  [unwired: 3 in, 2 out]
                        n137 = Open VI Reference(type specifier VI Refnum (for type only)=refnum<vi> refnum ("类型说明符VI引用句柄（仅用于类型）"), vi path=w317, options=128 ("选项")) -> (vi reference=w318:refnum<vi>, error out=w314:errorcluster)  [unwired: 3 in]
                        n138 = call-by-ref "开始异步调用"(reference=w318, error in=w314, "队列输入"=w309, "氨氮"=w308, "氨氮量程切换"=w306, "总磷"=w307, "总磷量程切换"=w305) -> (reference out=w316:refnum<vi>, error out=w315:errorcluster)  [unwired: 8 in, 3 out]
                        n139 = Close Reference(reference=w316, error in (no error)=w315) -> ()  [unwired: 1 out]
                      }
                    }
                    n140 = First Call?() -> (First Call?: T/F=w302:bool)
                    n141 = Select(t=FALSE, s=w302, f=TRUE) -> (s? t:f=w299:bool)
                  }
                }
                n142 = vi-ref "CODCr微站质控流程 (子VI).vi"() -> (w241:refnum<vi>)
                n143 = property class="VI"(reference=w241) -> ("Name"=w242:string, "Exec.State"=w243:T4)  [unwired: 1 in, 2 out]
                n144 = case shown="\"Idle\"" w243 {
                  tunnel: w242 -> [_ w269]
                  tunnel: [_ w264] -> w239
                  tunnel: w240 -> [_ w263]
                  frame "Bad", Default {
                  }
                  frame "Idle" {
                    n145 = First Call?() -> (First Call?: T/F=w268:bool)
                    n146 = case shown="真" w268 {
                      tunnel: w269 -> [_ w277]
                      tunnel: w263 -> [_ w270]
                      frame False {
                      }
                      frame True {
                        n147 = Open VI Reference(type specifier VI Refnum (for type only)=refnum<vi> refnum ("类型说明符VI引用句柄（仅用于类型）"), vi path=w277, options=128 ("选项")) -> (vi reference=w271:refnum<vi>, error out=w274:errorcluster)  [unwired: 3 in]
                        n148 = call-by-ref "开始异步调用"(reference=w271, error in=w274, "COD"=w270) -> (reference out=w276:refnum<vi>, error out=w275:errorcluster)  [unwired: 9 in, 2 out]
                        n149 = Close Reference(reference=w276, error in (no error)=w275) -> ()  [unwired: 1 out]
                      }
                    }
                    n150 = First Call?() -> (First Call?: T/F=w267:bool)
                    n151 = Select(t=FALSE, s=w267, f=TRUE) -> (s? t:f=w264:bool)
                  }
                }
                n152 = Compound Arithmetic op=AND ("复合运算")(w252, w259, w245, w239) -> (w262:bool)
              }
            }
            n153 = Select(t=enum16{"初始化", "采配水启动", "等待", "配水", "排水", "结束"}."排水" ("枚举"), s=w226, f=w230) -> (s? t:f=w229:enum16{"初始化", "采配水启动", "等待", "配水", "排水", "结束"})
          }
          frame "排水" {
            n154 = Enqueue Element At Opposite End(queue=w327, element=T2 {"命令"="单个写入", {"starting address"=303, "holding register value"=1}} ("元素")) -> ()  [unwired: 2 in, 3 out]
            n155 = Increment(x=w326) -> (x+1=w325:enum16{"初始化", "采配水启动", "等待", "配水", "排水", "结束"})
          }
          frame "结束" {
            n156 = Increment(x=w331) -> (x+1=w330:enum16{"初始化", "采配水启动", "等待", "配水", "排水", "结束"})
          }
        }
        "枚举" <- w193
        n157 = Wait (ms)(milliseconds to wait=u32 1000 ("等待时间（毫秒）")) -> ()  [unwired: 1 out]
        n158 = global write "质控测完标志全局 1.vi" "质控流程中"(TRUE ("质控流程中")) -> ()
        n159 = Get Notifier Status(notifier=w189) -> (notifier out=w188:refnum<notifier>, current notification=w186:bool)  [unwired: 1 in, 3 out]
        n160 = Or(x=w186, y=w187) -> (x .or. y?=w185:bool)
        n161 = case shown="真" w185 {
          frame False {
          }
          frame True {
            w196 = FALSE ("质控流程中")
            n162 = global write "质控测完标志全局 1.vi" "质控流程中"(w196) -> ()
            n163 = global write "质控测完标志全局 1.vi" "COD加标回收测完标志"(w196) -> ()
            n164 = global write "质控测完标志全局 1.vi" "总氮加标回收测完标志"(w196) -> ()
            n165 = global write "质控测完标志全局 1.vi" "氨氮加标回收测完标志"(w196) -> ()
            n166 = global write "质控测完标志全局 1.vi" "总磷加标回收测完标志"(w196) -> ()
          }
        }
      }
      n167 = Cancel Notification(0:w173) -> (8:w172:refnum<notifier>)  [unwired: 1 in, 2 out]
      n168 = Release Notifier(notifier=w172) -> ()  [unwired: 2 in, 3 out]
    }
  }
